vi "SPI Scripting.Create and Place IO Nodes.vi"(5 "Device Information":T1={"Number of Channels"=1, "Device Alias"="", "Device Icon Name"=[]}, 7 "Current Bus Path":path=path "D:/Documents/Projects/SPIAPI/IOEngineCode/Initialize Node Resources.vi", 8 "error in":errorcluster, 9 "Path to Analog Node Template":string="IONode\\Analog Input Node x.vi", 10 "Values for Naming":T2={"Bus Number"=1, "Device Number"=1, "Channel Number"=1} {"Channel Number" min=1 step=1; "Device Number" min=1 step=1; "Bus Number" min=1 step=1}, 11 "Virtual Folder":refnum<vi>) -> (0 "error out":errorcluster, 2 "Path to New Node":path, 3 "Path to IO Node":path=path "D:/Documents/Projects/SPIAPI/IOEngineCode/Initialize Node Resources.vi")   [LabVIEW 2014, in "Initialization and IO Node Scripting.lvlib"]
uses:
  Initialization and IO Node Scripting.lvlib
  State Machine/Controls/Values for Naming.ctl
  State Machine/Controls/Device Information.ctl
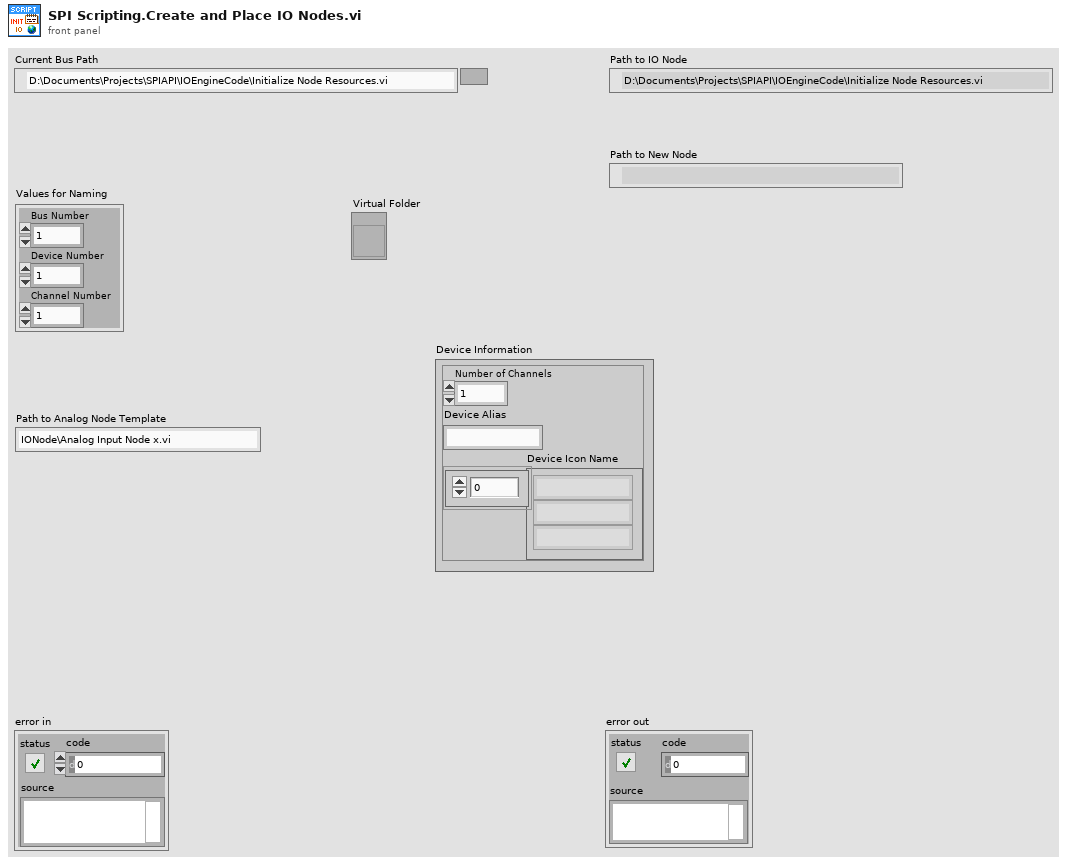
[diagram p1: front panel]
types:
  T1 = typedef "Device Information.ctl" = cluster{"Number of Channels":i32, "Device Alias":string, "Device Icon Name":string[]}
  T2 = typedef "Initialization and IO Node Scripting.lvlib/Values for Naming.ctl" = cluster{"Bus Number":i32, "Device Number":i32, "Channel Number":i32}
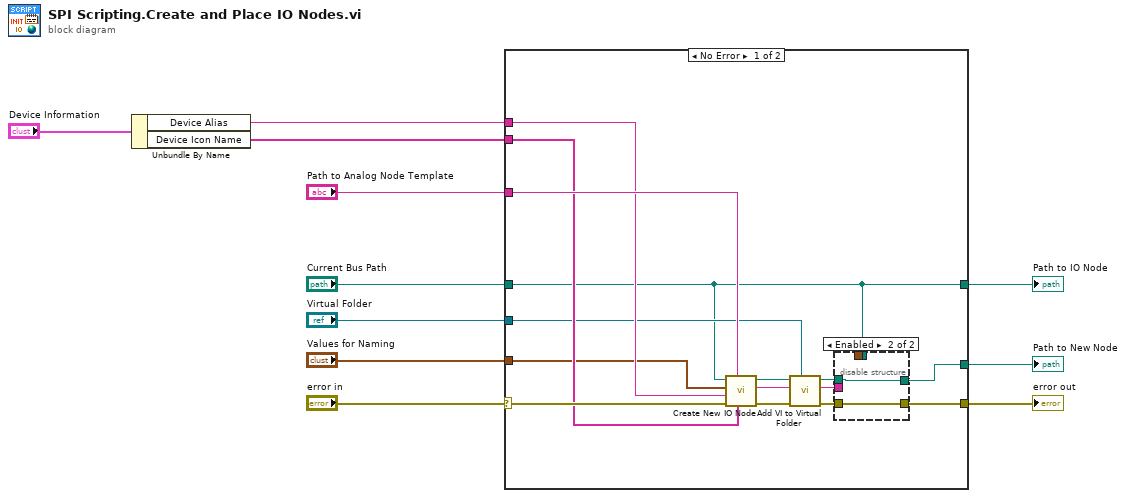
[diagram p0: block diagram]
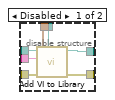
[diagram p2: hidden frame]
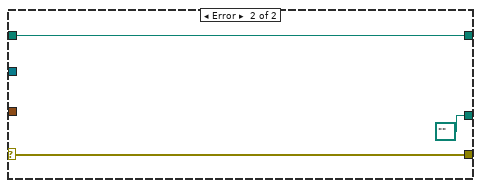
[diagram p3: hidden frame]
diagram:
  n1 = Unbundle By Name("Device Information") -> ("Device Alias"=w2:string, "Device Icon Name"=w3:string[])
  n2 = case shown="No Error" "error in" {
    selector: "error in" -> [w26 w38]
    tunnel: "Current Bus Path" -> [w15 w37]
    tunnel: [w14 w38] -> w9
    tunnel: [w15 w37] -> w8
    tunnel: "Virtual Folder" -> [w19 _]
    tunnel: "Values for Naming" -> [w13 _]
    tunnel: "Path to Analog Node Template" -> [w25 _]
    tunnel: w2 -> [w24 _]
    tunnel: w3 -> [w23 _]
    tunnel: [w12 path "" ("Path to VI")] -> w1
    frame No Error {
      n3 = call "Create New IO Node.vi"("Device Icon Name"=w23, "Path to Analog Node Template"=w25, "error in"=w26, "Device Alias"=w24, "Values for Naming"=w13, "Path to IO Node"=w15) -> ("error out"=w22:errorcluster, "IO Node Name"=w21:string, "Path to new IO Node"=w20:path)  [unwired: 3 in]
      n4 = call "Add VI to Virtual Folder.vi"("Virtual Folder"=w19, "error in"=w22, "VI Name"=w21, "Path to VI"=w20) -> ("error out"=w18:errorcluster, "VI Name"=w17:string, "Path to VI"=w16:path)  [unwired: 5 in]
      n5 = disable-structure shown="Enabled" {
        disable-tunnel: w18 -> [w33 w34]
        disable-tunnel: w17 -> [w32 _]
        disable-tunnel: w16 -> [w31 w35]
        disable-tunnel: w15 -> [w30 _]
        disable-tunnel: [w29 w34] -> w14
        disable-tunnel: [w28 w35] -> w12
        disable-tunnel: _ -> [w27 _]
        frame Disabled {
          n6 = call "Add VI to Library.vi"("Current Bus Path"=w30, "error in"=w33, "Bus Number"=w27, "VI Name"=w32, "Path to new VI"=w31) -> ("error out"=w29:errorcluster, "Path to new IO Node"=w28:path)  [unwired: 5 in]
        }
        frame Enabled {
        }
      }
    }
    frame Error {
    }
  }
  "error out" <- w9
  "Path to IO Node" <- w8
  "Path to New Node" <- w1
